vi "COM_FGET.vi"(11 "limit":i32=200) -> (2 "getString":string, 3 "return":i32)   [LabVIEW 2016]
panel:
  out "error out":errorcluster
  out "Numeric":i32
  out "read buffer 2":string
  out "read buffer":string
  out "length":i32
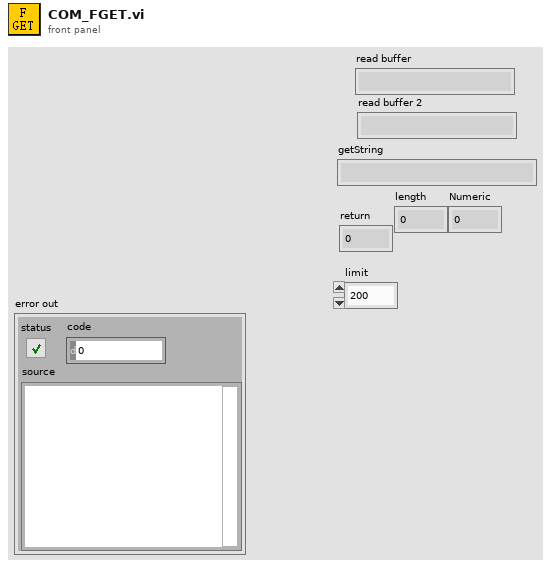
[diagram p1: front panel]
types:
  T1 = enum16{"initial", "write", "read", "release", "change"}
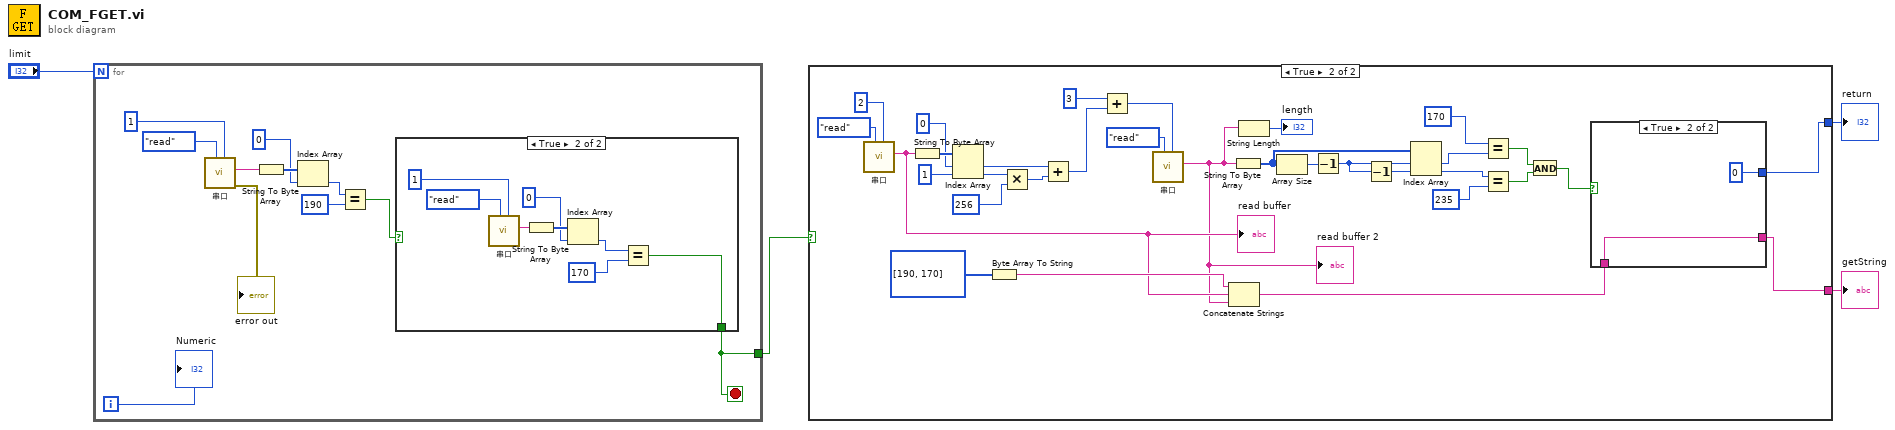
[diagram p0: block diagram]
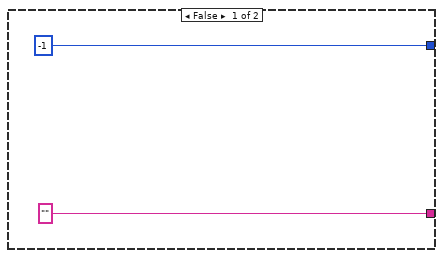
[diagram p2: hidden frame]
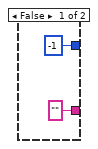
[diagram p3: hidden frame]
diagram:
  n1 = for {
    N: "limit" -> [_]
    tunnel: [w7] -> w3
    i -> [w6]
    stop <- w7 stop-if-true
    n2 = call "串口.vi"("byte count"=u32 1, "case"=T1."read") -> ("error out"=→"error out":errorcluster, "read buffer"=w13:string)  [unwired: 6 in, 2 out]
    n3 = String To Byte Array(string=w13) -> (unsigned byte array=w12:u8[])
    n4 = Index Array(array=w12, index=0) -> (element=w10:u8)
    n5 = Equal?(x=w10, y=u8 190) -> (x = y?=w8:bool)
    n6 = case shown="True" w8 {
      selector: w8 -> [w16 _]
      tunnel: [w16 w17] -> w7
      frame False {
      }
      frame True {
        n7 = call "串口.vi"("byte count"=u32 1, "case"=T1."read") -> ("read buffer"=w21:string)  [unwired: 6 in, 3 out]
        n8 = String To Byte Array(string=w21) -> (unsigned byte array=w22:u8[])
        n9 = Index Array(array=w22, index=0) -> (element=w19:u8)
        n10 = Equal?(x=w19, y=u8 170) -> (x = y?=w17:bool)
      }
    }
    "Numeric" <- w6
  }
  n11 = case shown="True" w3 {
    tunnel: ["" w33] -> w2
    tunnel: [-1 w32] -> w1
    frame False {
    }
    frame True {
      n12 = call "串口.vi"("byte count"=u32 2, "case"=T1."read") -> ("read buffer"=w31:string)  [unwired: 6 in, 3 out]
      "read buffer" <- w31
      n13 = String To Byte Array(string=w31) -> (unsigned byte array=w56:u8[])
      n14 = Index Array(array=w56, index #1=0 ("index"), index #2=1 ("index")) -> (element #1=w50:u8, element #2=w53:u8)
      n15 = Byte Array To String(unsigned byte array=u8[] [190, 170]) -> (string=w46:string)
      n16 = Multiply(x=w53, y=u16 256) -> (x*y=w51:u16)
      n17 = Add(x=w50, y=w51) -> (x+y=w48:u16)
      n18 = Add(x=u16 3, y=w48) -> (x+y=w29:u16)
      n19 = call "串口.vi"("byte count"=w29, "case"=T1."read") -> ("read buffer"=w28:string)  [unwired: 6 in, 3 out]
      "read buffer 2" <- w28
      n20 = Concatenate Strings(w46, w31, w28) -> (w34:string)
      n21 = String To Byte Array(string=w28) -> (unsigned byte array=w42:u8[])
      n22 = String Length(string=w28) -> (length=→"length":i32)
      n23 = Array Size(array=w42) -> (size(s)=w45:i32)
      n24 = Decrement(x=w45) -> (x-1=w44:i32)
      n25 = Decrement(x=w44) -> (x-1=w43:i32)
      n26 = Index Array(array=w42, index #1=w44, index #2=w43) -> (element #1=w41:u8, element #2=w39:u8)
      n27 = Equal?(x=u8 170, y=w41) -> (x = y?=w37:bool)
      n28 = Equal?(x=w39, y=u8 235) -> (x = y?=w36:bool)
      n29 = And(x=w37, y=w36) -> (x .and. y?=w35:bool)
      n30 = case shown="True" w35 {
        tunnel: w34 -> [_ w62]
        tunnel: ["" w62] -> w33
        tunnel: [-1 0] -> w32
        frame False {
        }
        frame True {
        }
      }
    }
  }
  "getString" <- w2
  "return" <- w1
